vi "current (SubVI).vi"(7 "Reset":bool, 8 "Max Current B":dbl, 9 "Max Current A":dbl, 10 "Array":bool[](array[boolean]), 11 "Current":T5={"Current dc A"=0.0, "Current dc B"=0.0, "Frequency A"=0.0, "Frequency B"=0.0, "Current hi A"=0.0, "Current hi B"=0.0, "Current low A"=0.0, "Current low B"=0.0, "Focal Power A"=3.0, "Temperature high A"=20.0, "Temperature low A"=45.0} {"Current dc A" scale=-200.0..200.0 scale format="%#_5g"; "Current dc B" scale=-200.0..200.0 scale format="%#_5g"; "Frequency A" scale=0.1..1000.0; "Frequency B" scale=0.1..1000.0; "Current hi A" scale=-200.0..200.0 scale format="%#_5g"; "Current hi B" scale=-200.0..200.0 scale format="%#_5g"; "Current low A" scale=-200.0..200.0 scale format="%#_5g"; "Current low B" scale=-200.0..200.0 scale format="%#_5g"; "Focal Power A" scale=-5.0..10.0 scale format="%#_5g"; "Temperature high A" scale=10.0..100.0; "Temperature low A" scale=10.0..100.0}) -> (0 "command":string[](array[string]))   [LabVIEW 2013]
doc: "This VI builds the command strings for changes of current"
uses:
  03 Type Def & Global/Slider.ctl
  03 Type Def & Global/Slider Freq.ctl
  03 Type Def & Global/Slider Focal Power.ctl
  03 Type Def & Global/Slider Temperature.ctl
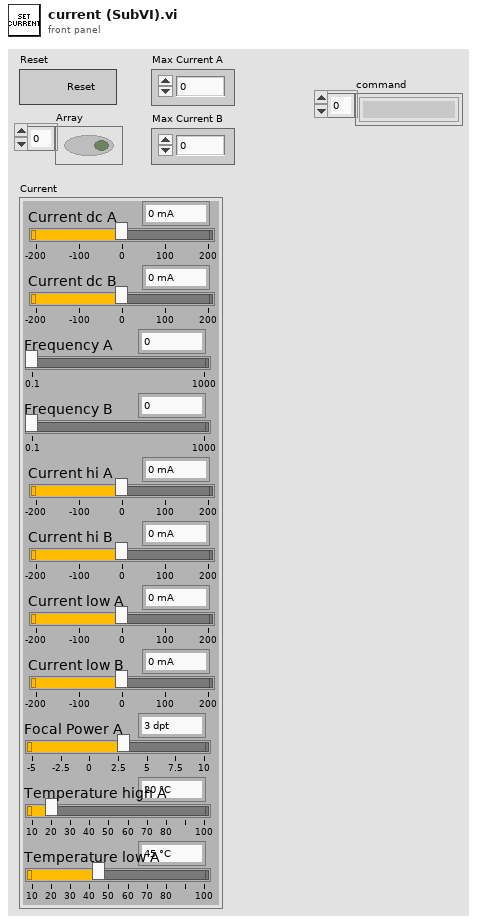
[diagram p1: front panel]
types:
  T1 = typedef "Slider.ctl" = dbl
  T2 = typedef "Slider Freq.ctl" = dbl
  T3 = typedef "Slider Focal Power.ctl" = dbl
  T4 = typedef "Slider Temperature.ctl" = dbl
  T5 = cluster{"Current dc A":T1, "Current dc B":T1, "Frequency A":T2, "Frequency B":T2, "Current hi A":T1, "Current hi B":T1, "Current low A":T1, "Current low B":T1, "Focal Power A":T3, "Temperature high A":T4, "Temperature low A":T4}
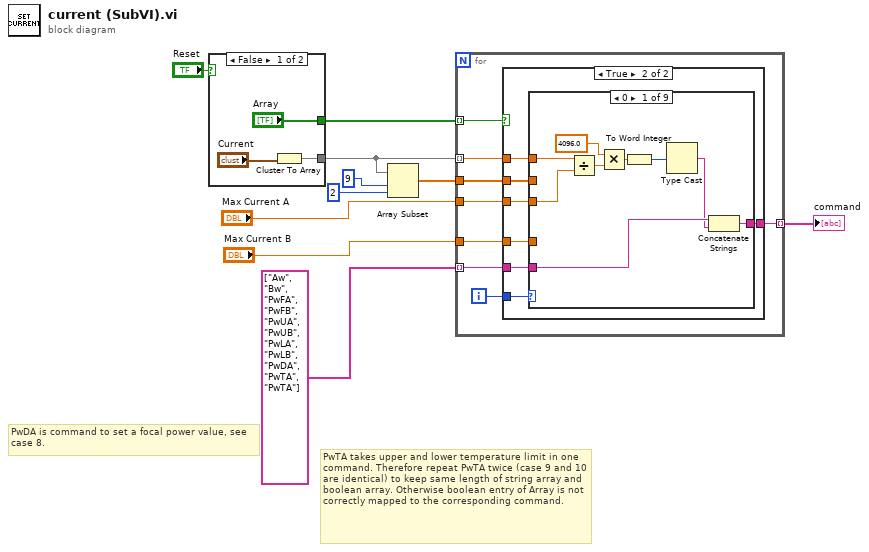
[diagram p0: block diagram]
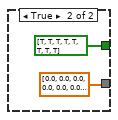
[diagram p2: hidden frame]
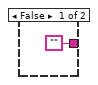
[diagram p3: hidden frame]
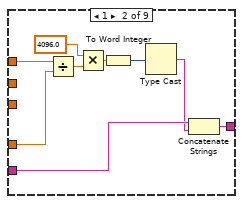
[diagram p4: hidden frame]
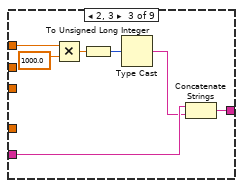
[diagram p5: hidden frame]
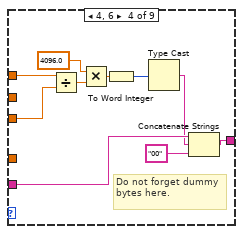
[diagram p6: hidden frame]
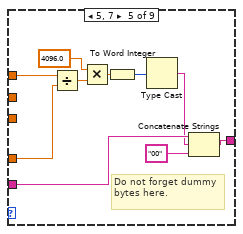
[diagram p7: hidden frame]
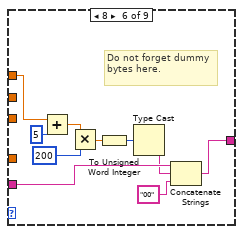
[diagram p8: hidden frame]
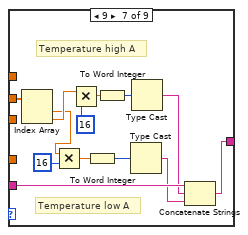
[diagram p9: hidden frame]
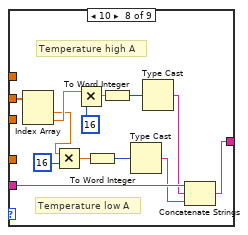
[diagram p10: hidden frame]
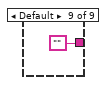
[diagram p11: hidden frame]
diagram:
  # "PwDA is command to set a focal power value, see case 8."
  # "PwTA takes upper and lower temperature limit in one command. Therefore repeat PwTA twice (case 9 and 10 are identical) to keep same length of string array and boolean array. Otherwise boolean entry of Array is not correctly mapped to the corresponding command."
  n1 = case shown="False" "Reset" {
    tunnel: ["Array" bool[] [TRUE, TRUE, TRUE, TRUE, TRUE, TRUE, TRUE, TRUE] ("Array 2")] -> w10
    tunnel: [w12 dbl[] [0.0, 0.0, 0.0, 0.0, 0.0, 0.0, 0.0, 0.0]] -> w4
    frame False {
      n2 = Cluster To Array(cluster="Current") -> (array=w12:T4[])
    }
    frame True {
    }
  }
  n3 = Array Subset(array=w4, index=9, length=2 ("index")) -> (w1:T4[])
  n4 = for {
    tunnel: w10 -> [w19] mode=indexing
    tunnel: w4 -> [w23] mode=indexing
    tunnel: string[] ["Aw", "Bw", "PwFA", "PwFB", "PwUA", "PwUB", "PwLA", "PwLB", "PwDA", "PwTA", "PwTA"] -> [w22] mode=indexing
    tunnel: [w20] -> w8 mode=indexing
    tunnel: "Max Current A" -> [w18]
    tunnel: "Max Current B" -> [w17]
    tunnel: w1 -> [w16]
    i -> [w21]
    n5 = case shown="True" w19 {
      tunnel: w23 -> [_ w30]
      tunnel: w22 -> [_ w29]
      tunnel: w21 -> [_ w31]
      tunnel: ["" w28] -> w20
      tunnel: w18 -> [_ w27]
      tunnel: w17 -> [_ w26]
      tunnel: w16 -> [_ w25]
      frame False {
      }
      frame True {
        n6 = case shown="0" w31 {
          tunnel: w30 -> [w34 w49 w56 w59 w69 w79 _ _ _]
          tunnel: w29 -> [w40 w46 w53 w66 w76 w83 w97 w110 _]
          tunnel: [w39 w45 w54 w65 w75 w81 w96 w109 ""] -> w28
          tunnel: w27 -> [w33 _ _ w58 _ _ _ _ _]
          tunnel: w26 -> [_ w44 _ _ w68 _ _ _ _]
          tunnel: w25 -> [_ _ _ _ _ _ w95 w108 _]
          frame 0 {
            n7 = Divide(x=w34, y=w33) -> (x/y=w38:T4)
            n8 = Multiply(x=4096.0, y=w38) -> (x*y=w36:T4)
            n9 = To Word Integer(number=w36) -> (16bit integer=w35:i16)
            n10 = Type Cast(x=w35) -> (*(type *) &x=w32:string)  [unwired: 1 in]
            n11 = Concatenate Strings(w40, w32) -> (w39:string)
          }
          frame 1 {
            n12 = Divide(x=w49, y=w44) -> (x/y=w48:T4)
            n13 = Multiply(x=4096.0, y=w48) -> (x*y=w43:T4)
            n14 = To Word Integer(number=w43) -> (16bit integer=w41:i16)
            n15 = Type Cast(x=w41) -> (*(type *) &x=w42:string)  [unwired: 1 in]
            n16 = Concatenate Strings(w46, w42) -> (w45:string)
          }
          frame 2, 3 {
            n17 = Multiply(x=w56, y=1000.0) -> (x*y=w52:T4)
            n18 = To Unsigned Long Integer(number=w52) -> (unsigned 32bit integer=w51:u32)
            n19 = Type Cast(x=w51) -> (*(type *) &x=w50:string)  [unwired: 1 in]
            n20 = Concatenate Strings(w53, w50) -> (w54:string)
          }
          frame 4, 6 {
            # "Do not forget dummy bytes here."
            n21 = Divide(x=w59, y=w58) -> (x/y=w63:T4)
            n22 = Multiply(x=4096.0, y=w63) -> (x*y=w61:T4)
            n23 = To Word Integer(number=w61) -> (16bit integer=w60:i16)
            n24 = Type Cast(x=w60) -> (*(type *) &x=w57:string)  [unwired: 1 in]
            n25 = Concatenate Strings(w66, w57, "00") -> (w65:string)
          }
          frame 5, 7 {
            # "Do not forget dummy bytes here."
            n26 = Divide(x=w69, y=w68) -> (x/y=w73:T4)
            n27 = Multiply(x=4096.0, y=w73) -> (x*y=w71:T4)
            n28 = To Word Integer(number=w71) -> (16bit integer=w70:i16)
            n29 = Type Cast(x=w70) -> (*(type *) &x=w67:string)  [unwired: 1 in]
            n30 = Concatenate Strings(w76, w67, "00") -> (w75:string)
          }
          frame 8 {
            # "Do not forget dummy bytes here."
            n31 = Add(x=w79, y=u16 5) -> (x+y=w85:T4)
            n32 = Multiply(x=w85, y=u16 200) -> (x*y=w78:T4)
            n33 = To Unsigned Word Integer(number=w78) -> (unsigned 16bit integer=w77:u16)
            n34 = Type Cast(x=w77) -> (*(type *) &x=w82:string)  [unwired: 1 in]
            n35 = Concatenate Strings(w83, w82, "00") -> (w81:string)
          }
          frame 9 {
            # "Temperature high A"
            # "Temperature low A"
            n36 = Index Array(array=w95) -> (element #1=w87:T4, element #2=w88:T4)  [unwired: 2 in]
            n37 = Multiply(x=w87, y=i16 16) -> (x*y=w91:T4)
            n38 = Multiply(x=w88, y=i16 16) -> (x*y=w94:T4)
            n39 = To Word Integer(number=w91) -> (16bit integer=w92:i16)
            n40 = To Word Integer(number=w94) -> (16bit integer=w93:i16)
            n41 = Type Cast(x=w92) -> (*(type *) &x=w90:string)  [unwired: 1 in]
            n42 = Type Cast(x=w93) -> (*(type *) &x=w89:string)  [unwired: 1 in]
            n43 = Concatenate Strings(w97, w89, w90) -> (w96:string)
          }
          frame 10 {
            # "Temperature high A"
            # "Temperature low A"
            n44 = Index Array(array=w108) -> (element #1=w100:T4, element #2=w101:T4)  [unwired: 2 in]
            n45 = Multiply(x=w100, y=i16 16) -> (x*y=w104:T4)
            n46 = Multiply(x=w101, y=i16 16) -> (x*y=w107:T4)
            n47 = To Word Integer(number=w104) -> (16bit integer=w105:i16)
            n48 = To Word Integer(number=w107) -> (16bit integer=w106:i16)
            n49 = Type Cast(x=w105) -> (*(type *) &x=w103:string)  [unwired: 1 in]
            n50 = Type Cast(x=w106) -> (*(type *) &x=w102:string)  [unwired: 1 in]
            n51 = Concatenate Strings(w110, w102, w103) -> (w109:string)
          }
          frame Default {
          }
        }
      }
    }
  }
  "command" <- w8
